vi "NetComm_getMatchInfo.vi"(8 "error in (no error)":errorcluster) -> (0 "error out":errorcluster, 1 "Game Specific Data":string, 2 "Match Type":T1, 3 "Event Name":string, 4 "Replay Number":u16, 5 "Match Number":u16)   [LabVIEW 2017]
uses:
  <vilib>/Rock Robotics/SystemInterfaces/NetworkCommunication/NetComm_MatchType.ctl
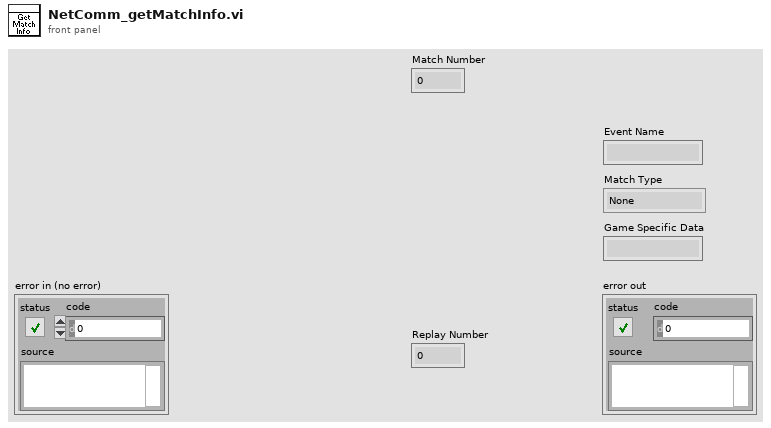
[diagram p1: front panel]
types:
  T1 = typedef "NetComm_MatchType.ctl" = enum32{"None", "Practice", "Qualification", "Elimination"}
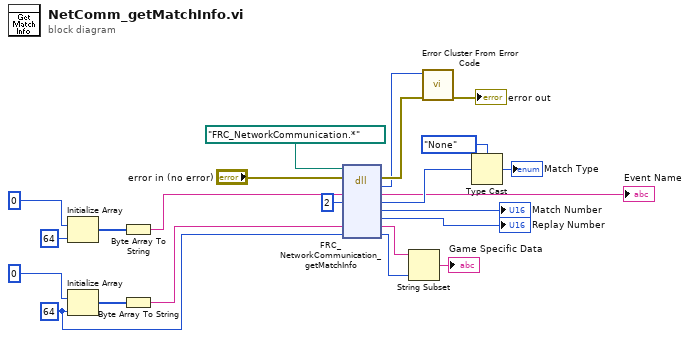
[diagram p0: block diagram]
diagram:
  w5 = 64 ("dimension size")
  n1 = Initialize Array(u8 0, 64 ("dimension size")) -> (w16:u8[])
  n2 = Initialize Array(u8 0, w5) -> (w8:u8[])
  n3 = Byte Array To String(unsigned byte array=w16) -> (string=w15:string)
  n4 = Byte Array To String(unsigned byte array=w8) -> (string=w6:string)
  n5 = dll-call lib="?" fn="FRC_NetworkCommunication_getMatchInfo"(path in=path "FRC_NetworkCommunication.*", error in="error in (no error)", "eventName"=w15, "matchType"=u16 2, "gameSpecificMessage"=w6, "gameSpecificMessageSize"=w5) -> (error out=w21:errorcluster, "return type"=w20:i32, "eventName"=→"Event Name":string, "matchType"=w13:i32, "matchNumber"=→"Match Number":u16, "replayNumber"=→"Replay Number":u16, "gameSpecificMessage"=w4:string, "gameSpecificMessageSize"=w3:u8)  [unwired: 3 in, 1 out]
  n6 = String Subset(string=w4, length (rest)=w3) -> (substring=→"Game Specific Data":string)  [unwired: 1 in]
  n7 = call <vilib>:"Error Cluster From Error Code.vi"("error in (no error)"=w21, "error code (0)"=w20) -> ("error out"=→"error out":errorcluster)  [unwired: 7 in]
  n8 = Type Cast(type=NetComm_MatchType."None", x=w13) -> (*(type *) &x=→"Match Type":T1)
